vi "Create Window.vi"(8 "error in (no error)":errorcluster, 10 "Window":refnum<vi>) -> (0 "error out":errorcluster, 3 "Window out":refnum<class "Window.lvclass">)   [LabVIEW 2015, in "IBEX Device.lvlib" / "Window.lvclass"]
doc: "Creates a Window.lvclass object."
uses:
  Window.lvclass
  Window.lvclass/Window.ctl
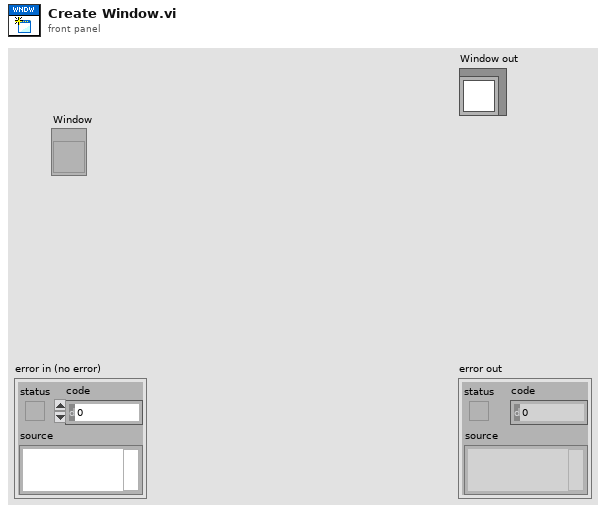
[diagram p1: front panel]
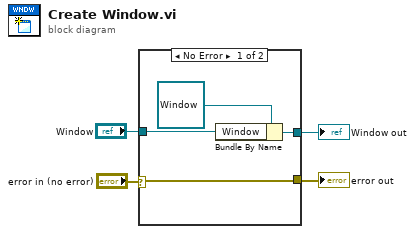
[diagram p0: block diagram]
diagram:
  n1 = case shown="No Error" "error in (no error)" {
    selector: "error in (no error)" -> [w6 w9]
    tunnel: [w8 _] -> w4
    tunnel: "Window" -> [w7 _]
    tunnel: [w6 w9] -> w2
    frame No Error {
      n2 = Bundle By Name(cluster=refnum<class "Window.lvclass"> refnum ("Window in"), "Window"=w7) -> (w8:refnum<class "Window.lvclass">)
    }
    frame Error {
    }
  }
  "error out" <- w2
  "Window out" <- w4
